vi "xmlFeature2.vi"(10 "Array":string[][](array[string]), 11 "Numeric":i32) -> ()   [LabVIEW 2018]
uses:
  Global Variables.vi
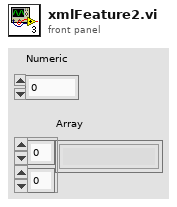
[diagram p1: front panel]
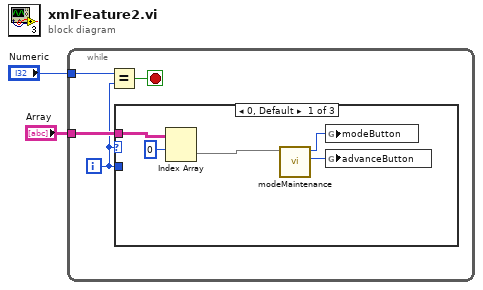
[diagram p0: block diagram]
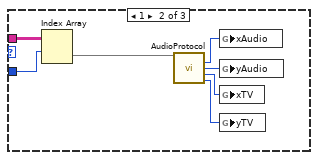
[diagram p2: hidden frame]
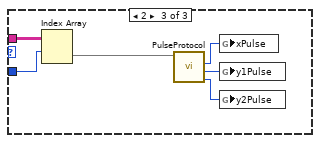
[diagram p3: hidden frame]
diagram:
  n1 = while {
    tunnel: "Numeric" -> [w5]
    tunnel: "Array" -> [w4]
    i -> [w3]
    stop <- w6 stop-if-true
    n2 = Equal?(x=w5, y=w3) -> (x = y?=w6:bool)
    n3 = case shown="0, Default" w3 {
      tunnel: w4 -> [w9 w13 w20]
      tunnel: w3 -> [_ w12 w21]
      frame 0, Default {
        n4 = Index Array(array=w9, index (row)=0) -> (element=w8:string[])  [unwired: 1 in]
        n5 = call "modeMaintenance.vi"("Array"=w8) -> ("advanceButton"=w11:i32, "modeButton"=w10:i32)  [unwired: 9 in]
        n6 = global write "Global Variables.vi" "modeButton"(w10) -> ()
        n7 = global write "Global Variables.vi" "advanceButton"(w11) -> ()
      }
      frame 1 {
        n8 = Index Array(array=w13, index (row)=w12) -> (element=w14:string[])  [unwired: 1 in]
        n9 = call "AudioProtocol.vi"("Array"=w14) -> ("xAudio"=w15:i32, "yAudio"=w16:i32, "xTV"=w17:i32, "yTV"=w18:i32)  [unwired: 10 in, 1 out]
        n10 = global write "Global Variables.vi" "xAudio"(w15) -> ()
        n11 = global write "Global Variables.vi" "yAudio"(w16) -> ()
        n12 = global write "Global Variables.vi" "xTV"(w17) -> ()
        n13 = global write "Global Variables.vi" "yTV"(w18) -> ()
      }
      frame 2 {
        n14 = Index Array(array=w20, index (row)=w21) -> (element=w19:string[])  [unwired: 1 in]
        n15 = call "PulseProtocol.vi"("Array"=w19) -> ("y2Pulse"=w24:i32, "y1Pulse"=w23:i32, "xPulse"=w22:i32)  [unwired: 7 in, 1 out]
        n16 = global write "Global Variables.vi" "xPulse"(w22) -> ()
        n17 = global write "Global Variables.vi" "y1Pulse"(w23) -> ()
        n18 = global write "Global Variables.vi" "y2Pulse"(w24) -> ()
      }
    }
  }
